vi "UTIL State Dependent-Random Walk.vi"(3 "Boolean":bool, 4 "Numeric":dbl, 5 "Parameters Out":dbl[](array[numeric]), 6 "Temperature Units (C)":u16) -> (0 "Target Temp":dbl, 1 "Parameters Out":dbl[](array[numeric]), 2 "Q":dbl)   [LabVIEW 2010]
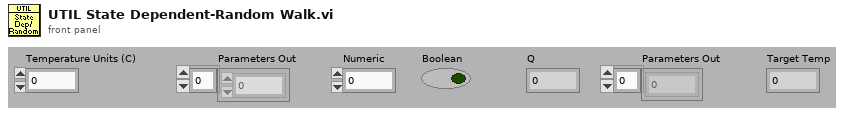
[diagram p1: front panel]
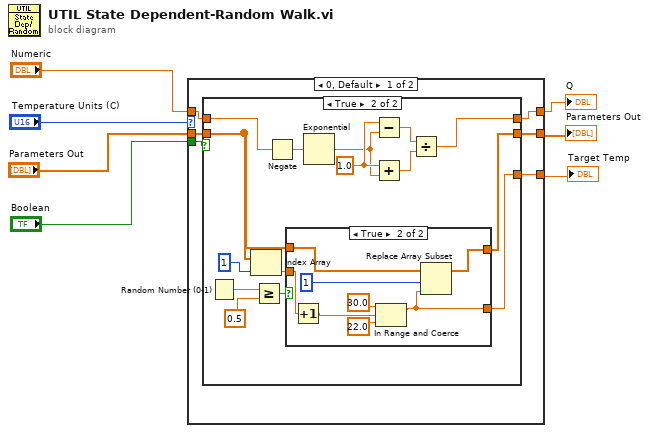
[diagram p0: block diagram]
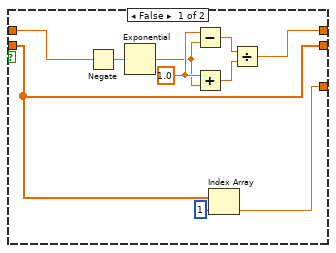
[diagram p2: hidden frame]
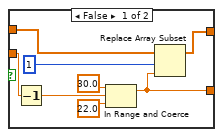
[diagram p3: hidden frame]
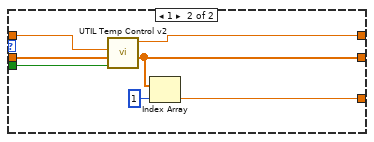
[diagram p4: hidden frame]
diagram:
  n1 = case shown="0, Default" "Temperature Units (C)" {
    tunnel: "Boolean" -> [w10 w61]
    tunnel: [w12 w56] -> w2
    tunnel: "Parameters Out" -> [w13 w60]
    tunnel: [w8 w59] -> w4
    tunnel: "Numeric" -> [w9 w58]
    tunnel: [w11 w55] -> w7
    frame 0, Default {
      n2 = case shown="True" w10 {
        tunnel: w13 -> [w23 w33]
        tunnel: [w23 w32] -> w12
        tunnel: [w21 w31] -> w11
        tunnel: w9 -> [w14 w24]
        tunnel: [w15 w25] -> w8
        frame False {
          w20 = 1.0 ("x")
          n3 = Negate(x=w14) -> (-x=w19:dbl)
          n4 = Exponential(1:w19) -> (0:w18:dbl)
          n5 = Subtract(x=w20, y=w18) -> (x-y=w17:dbl)
          n6 = Add(x=w20, y=w18) -> (x+y=w16:dbl)
          n7 = Index Array(array=w23, index=1) -> (element=w21:dbl)
          n8 = Divide(x=w17, y=w16) -> (x/y=w15:dbl)
        }
        frame True {
          w30 = 1.0 ("x")
          n9 = Random Number (0-1)() -> (number: 0 to 1=w38:dbl)
          n10 = Index Array(array=w33, index=1) -> (element=w35:dbl)
          n11 = Greater Or Equal?(x=w38, y=0.5) -> (x >= y?=w34:bool)
          n12 = Negate(x=w24) -> (-x=w29:dbl)
          n13 = case shown="True" w34 {
            tunnel: w35 -> [w46 w54]
            tunnel: w33 -> [w45 w53]
            tunnel: [w43 w51] -> w32
            tunnel: [w39 w47] -> w31
            frame False {
              n14 = Decrement(x=w46) -> (x-1=w40:dbl)
              n15 = In Range and Coerce(upper limit=30.0 ("element"), x=w40, lower limit=22.0 ("element")) -> (coerced(x)=w39:dbl)  [unwired: 1 out]
              n16 = Replace Array Subset(array=w45, new element=w39, index=1) -> (w43:dbl[])
            }
            frame True {
              n17 = Increment(x=w54) -> (x+1=w48:dbl)
              n18 = In Range and Coerce(upper limit=30.0 ("element"), x=w48, lower limit=22.0 ("element")) -> (coerced(x)=w47:dbl)  [unwired: 1 out]
              n19 = Replace Array Subset(array=w53, new element=w47, index=1) -> (w51:dbl[])
            }
          }
          n20 = Exponential(1:w29) -> (0:w28:dbl)
          n21 = Subtract(x=w30, y=w28) -> (x-y=w27:dbl)
          n22 = Add(x=w30, y=w28) -> (x+y=w26:dbl)
          n23 = Divide(x=w27, y=w26) -> (x/y=w25:dbl)
        }
      }
    }
    frame 1 {
      n24 = call "UTIL Temp Control v2.vi"("Evaluate"=w61, "Parameters In"=w60, "Sleep Wake Ratio"=w58) -> ("Parameters Out"=w56:dbl[], "Q"=w59:dbl)  [unwired: 3 in]
      n25 = Index Array(array=w56, index=1) -> (element=w55:dbl)
    }
  }
  "Target Temp" <- w7
  "Q" <- w4
  "Parameters Out" <- w2
